vi "Close Subpanel.vi"(8 "error in (no error)":errorcluster, 11 "SubPanel in":refnum<vi>) -> (0 "error out":errorcluster, 3 "SubPanel out":refnum<vi>)   [LabVIEW 2016]
doc: "This VI closes the VI in a subpanel, closes the reference to it and removes it from the subpanel."
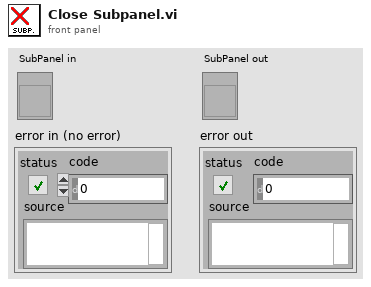
[diagram p1: front panel]
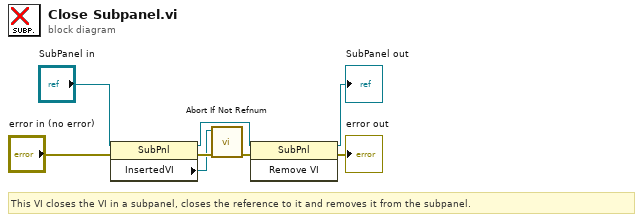
[diagram p0: block diagram]
diagram:
  # "This VI closes the VI in a subpanel, closes the reference to it and removes it from the subpanel."
  n1 = property class="SubPnl"(reference="SubPanel in", error in="error in (no error)") -> (reference out=w6:refnum<vi>, error out=w4:errorcluster, "InsertedVI"=w2:refnum<vi>)
  n2 = call "Abort If Not Refnum.vi"("error in (no error)"=w4, "VI in"=w2) -> ("error out"=w5:errorcluster)  [unwired: 9 in]
  n3 = invoke class="SubPnl" method="Remove VI"(reference=w6, error in=w5) -> (reference out=→"SubPanel out":refnum<vi>, error out=→"error out":errorcluster)  [unwired: 1 in, 1 out]
